vi "Apply Theme To Title.vi"(7 "Override Root With (Empty)":string, 8 "Error In":errorcluster, 9 "Window Element":T1, 10 "Title Ref":refnum<vi>, 11 "ini Theme in":refnum<class "ini Theme.lvclass">) -> (0 "Error Out":errorcluster, 3 "ini Theme out":refnum<class "ini Theme.lvclass">)   [LabVIEW 2021, in "Appearance Actor.lvlib" / "ini Theme.lvclass"]
doc: "Apply theme to a <B>Title</B> (String Reference). <B>Window Element</B> enum tells where it is on the window. <B>Override Root With</B> allows to override styling used for main window components."
uses:
  ini Theme.lvclass
  Generic Theme/API/Typedefs/Window Element--enum.ctl
  Generic Theme/API/Typedefs/Theme Control Property--enum.ctl
  ini Theme.lvclass/ini Theme.ctl
  f5176d82-9832-41ee-acb3-f85e09ee67a5.vi
  75531ee6-de61-497d-ad3a-faa2ff27009f.vi
  b8cf2edb-bf9c-49ba-affa-dd3e3f1f4187.vi
  478b1a93-bd91-4564-ac0e-3459a296c1aa.vi
  f5176d82-9832-41ee-acb3-f85e09ee67a5.vi/e124eda1-1651-4d76-919f-d33a8200b27b.vi
  f5176d82-9832-41ee-acb3-f85e09ee67a5.vi/2055fcb7-c480-499a-9c31-028cc01b484e.vi
  75531ee6-de61-497d-ad3a-faa2ff27009f.vi/e124eda1-1651-4d76-919f-d33a8200b27b.vi
  75531ee6-de61-497d-ad3a-faa2ff27009f.vi/2055fcb7-c480-499a-9c31-028cc01b484e.vi
  b8cf2edb-bf9c-49ba-affa-dd3e3f1f4187.vi/7b6ff018-fd93-4e92-b5eb-42dd48d1cdb9.vi
  b8cf2edb-bf9c-49ba-affa-dd3e3f1f4187.vi/6add14ee-ca76-441a-905a-1b37a406c8a7.vi
  478b1a93-bd91-4564-ac0e-3459a296c1aa.vi/e124eda1-1651-4d76-919f-d33a8200b27b.vi
  478b1a93-bd91-4564-ac0e-3459a296c1aa.vi/2055fcb7-c480-499a-9c31-028cc01b484e.vi
  Generic Theme/API/Utilities/Theme Entry Enum To String.vi
  Generic Theme/API/Constants/Default Entry Value--String.vi
  <vilib>/Utility/config.llb/Read Key.vi
  <vilib>/Utility/config.llb/Read Key (String).vi
  Generic Theme/API/Constants/Default Entry Value--U32.vi
  <vilib>/Utility/config.llb/Read Key (U32).vi
  <vilib>/Utility/config.llb/NI_LVConfig.lvlib
  Generic Theme/Generic Theme.lvclass
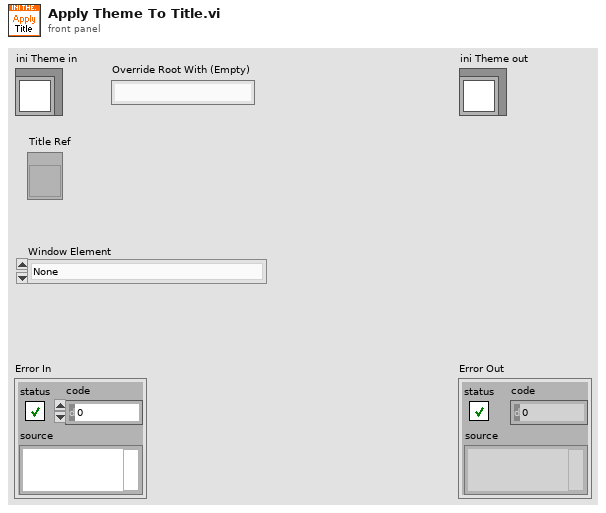
[diagram p1: front panel]
types:
  T1 = typedef "Appearance Actor.lvlib/Generic Theme.lvclass/Window Element--enum.ctl" = enum16{"None", "TB", "SM", "BP", "SB"}
  T2 = typedef "Appearance Actor.lvlib/Generic Theme.lvclass/Theme Control Property--enum.ctl" = enum16{"None", "Button.FalseFillColor", "Button.FalseOutlineColor", "Button.FalseToTrueFillColor", "Button.FalseToTrueOutlineColor", "Button.HoverFalseFillColor", "Button.HoverFalseOutlineColor", "Button.HoverTrueFillColor", "Button.HoverTrueOutlineColor", "Button.TrueFillColor", "Button.TrueOutlineColor", "Button.TrueToFalseFillColor", "Button.TrueToFalseOutlineColor", "CloseButton.FalseFillColor", "CloseButton.FalseOutlineColor", "CloseButton.FalseToTrueFillColor", "CloseButton.FalseToTrueOutlineColor", "CloseButton.HoverFalseFillColor", "CloseButton.HoverFalseOutlineColor", "CloseButton.HoverTrueFillColor", "CloseButton.HoverTrueOutlineColor", "CloseButton.TrueFillColor", "CloseButton.TrueOutlineColor", "CloseButton.TrueToFalseFillColor", "CloseButton.TrueToFalseOutlineColor", "Pane.Color", "Splitter.FillColor", "Splitter.OutlineColor", "Splitter.Size", "Title.Font.Color", "Title.Font.Family", "Title.Font.Size", "Title.Font.Style"}
  T3 = typedef "NI_LVConfig.lvlib/Config Data RefNum.ctl" = refnum<k1>
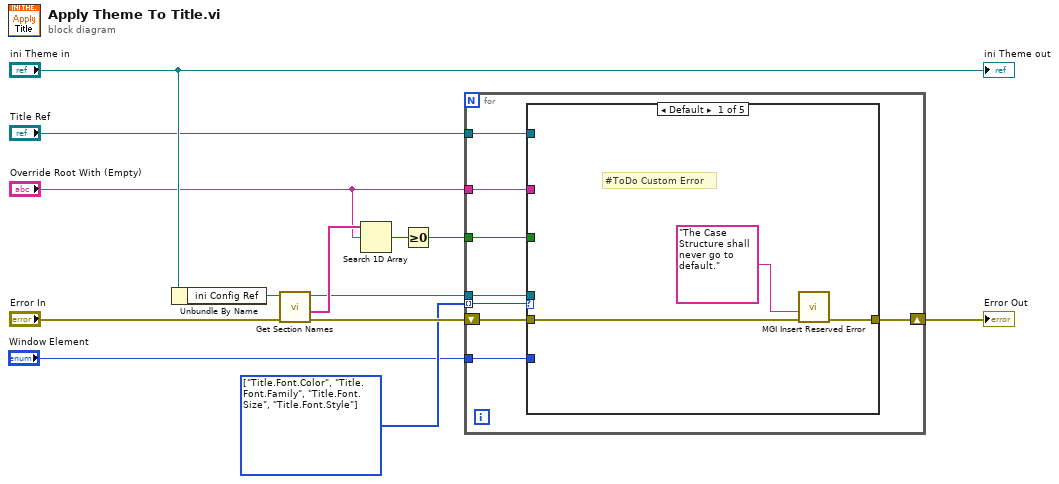
[diagram p0: block diagram]
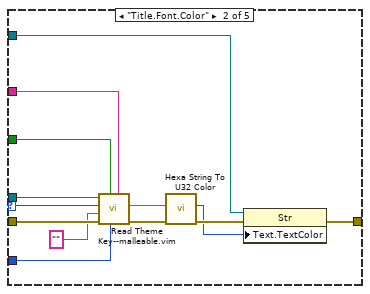
[diagram p2: hidden frame]
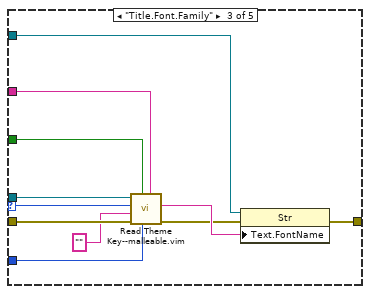
[diagram p3: hidden frame]
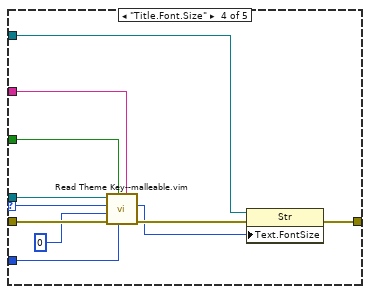
[diagram p4: hidden frame]
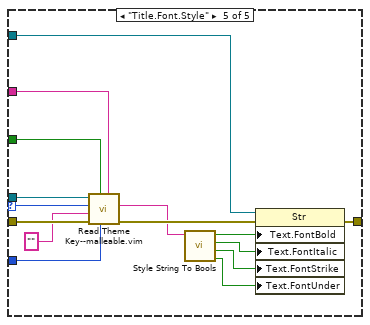
[diagram p5: hidden frame]
diagram:
  w2 = T2[] [enum."Title.Font.Color", enum."Title.Font.Family", enum."Title.Font.Size", enum."Title.Font.Style"] items=["None", "Button.FalseFillColor", "Button.FalseOutlineColor", "Button.FalseToTrueFillColor", "Button.FalseToTrueOutlineColor", "Button.HoverFalseFillColor", "Button.HoverFalseOutlineColor", "Button.HoverTrueFillColor", "Button.HoverTrueOutlineColor", "Button.TrueFillColor", "Button.TrueOutlineColor", "Button.TrueToFalseFillColor", "Button.TrueToFalseOutlineColor", "CloseButton.FalseFillColor", "CloseButton.FalseOutlineColor", "CloseButton.FalseToTrueFillColor", "CloseButton.FalseToTrueOutlineColor", "CloseButton.HoverFalseFillColor", "CloseButton.HoverFalseOutlineColor", "CloseButton.HoverTrueFillColor", "CloseButton.HoverTrueOutlineColor", "CloseButton.TrueFillColor", "CloseButton.TrueOutlineColor", "CloseButton.TrueToFalseFillColor", "CloseButton.TrueToFalseOutlineColor", "Pane.Color", "Splitter.FillColor", "Splitter.OutlineColor", "Splitter.Size", "Title.Font.Color", "Title.Font.Family", "Title.Font.Size", "Title.Font.Style"] ("Array")
  n1 = Unbundle By Name("ini Theme in") -> ("ini Config Ref"=w13:T3)
  n2 = call <vilib>:"Get Section Names.vi"("error in (no error)"="Error In", "refnum"=w13) -> ("error out"=w10:errorcluster, "section names"=w12:string[], "refnum out"=w4:T3)  [unwired: 7 in]
  n3 = Search 1D Array(1D array=w12, element="Override Root With (Empty)") -> (index of element=w11:i32)  [unwired: 1 in]
  n4 = Greater Or Equal To 0?(x=w11) -> (x >= 0?=w5:bool)
  n5 = for {
    shift-right: [w16] -> w8
    shift-left: w10 -> [w21]
    tunnel: "Override Root With (Empty)" -> [w20]
    tunnel: w5 -> [w19]
    tunnel: w4 -> [w18]
    tunnel: w2 -> [w17] mode=indexing
    tunnel: "Title Ref" -> [w15]
    tunnel: "Window Element" -> [w14]
    n6 = case shown="Default" w17 {
      selector: w17 -> [_ w33 w42 w54 w65]
      tunnel: w21 -> [w23 w34 w44 w56 w67]
      tunnel: w20 -> [_ w26 w38 w49 w60]
      tunnel: w19 -> [_ w31 w39 w50 w63]
      tunnel: w18 -> [_ w32 w45 w53 w64]
      tunnel: [w22 w36 w47 w58 w73] -> w16
      tunnel: w15 -> [_ w35 w46 w57 w72]
      tunnel: w14 -> [_ w25 w37 w48 w59]
      frame Default {
        # "#ToDo Custom Error"
        n7 = call <userlib>:"MGI Insert Reserved Error.vi"("Error In"=w23, "Error Description"="The Case Structure shall never go to default.") -> ("Error Out"=w22:errorcluster)  [unwired: 9 in]
      }
      frame "Title.Font.Color" {
        n8 = call "Read Theme Key--malleable.vim"("Section for Override (Empty)"=w26, "Window Element"=w25, "Can Be Overriden (F)"=w31, "Error In"=w34, "Data Type"="", "Theme Control Property"=w33, "ini Ref In"=w32) -> ("Error Out"=w29:errorcluster, "Value"=w28:string)  [unwired: 2 in, 1 out]
        n9 = call "Hexa String To U32 Color.vi"("8 Char Hexa String"=w28) -> ("U32 Color"=w27:u32)  [unwired: 10 in]
        n10 = property class="Str"(reference=w35, error in=w29, "Text.TextColor"=w27) -> (error out=w36:errorcluster)  [unwired: 1 out]
      }
      frame "Title.Font.Family" {
        n11 = call "Read Theme Key--malleable.vim"("Section for Override (Empty)"=w38, "Window Element"=w37, "Can Be Overriden (F)"=w39, "Error In"=w44, "Data Type"="", "Theme Control Property"=w42, "ini Ref In"=w45) -> ("Error Out"=w40:errorcluster, "Value"=w41:string)  [unwired: 2 in, 1 out]
        n12 = property class="Str"(reference=w46, error in=w40, "Text.FontName"=w41) -> (error out=w47:errorcluster)  [unwired: 1 out]
      }
      frame "Title.Font.Size" {
        n13 = call "Read Theme Key--malleable.vim"("Section for Override (Empty)"=w49, "Window Element"=w48, "Can Be Overriden (F)"=w50, "Error In"=w56, "Data Type"=u32 0, "Theme Control Property"=w54, "ini Ref In"=w53) -> ("Error Out"=w52:errorcluster, "Value"=w51:u32)  [unwired: 2 in, 1 out]
        n14 = property class="Str"(reference=w57, error in=w52, "Text.FontSize"=w51) -> (error out=w58:errorcluster)  [unwired: 1 out]
      }
      frame "Title.Font.Style" {
        n15 = call "Read Theme Key--malleable.vim"("Section for Override (Empty)"=w60, "Window Element"=w59, "Can Be Overriden (F)"=w63, "Error In"=w67, "Data Type"="" ("Default"), "Theme Control Property"=w65, "ini Ref In"=w64) -> ("Error Out"=w62:errorcluster, "Value"=w61:string)  [unwired: 2 in, 1 out]
        n16 = call "Style String To Bools.vi"("Style String"=w61) -> ("Underlined"=w68:bool, "Strikeout"=w69:bool, "Italic"=w70:bool, "Bold"=w71:bool)  [unwired: 7 in]
        n17 = property class="Str"(reference=w72, error in=w62, "Text.FontBold"=w71, "Text.FontItalic"=w70, "Text.FontStrike"=w69, "Text.FontUnder"=w68) -> (error out=w73:errorcluster)  [unwired: 1 out]
      }
    }
  }
  "Error Out" <- w8
  "ini Theme out" <- "ini Theme in"
